vi "Read Record.vi"(8 "error in (no error)":errorcluster, 11 "Configuration Database Actor in":refnum<class "Configuration Database Actor.lvclass">) -> (0 "error out":errorcluster, 3 "Configuration Database Actor out":refnum<class "Configuration Database Actor.lvclass">)   [LabVIEW 2022 SP3, in "Configuration Database Actor.lvlib" / "Configuration Database Actor.lvclass"]
uses:
  Configuration Database Actor.lvclass
  C:/Program Files/National Instruments/LabVIEW 2022/vi.lib/ActorFramework/Actor/Actor.lvclass
  <vilib>/ActorFramework/Actor/Actor.lvclass/Actor.ctl
  Configuration Database Actor.lvclass/Configuration Database Actor.ctl
  Interface Elevator/Interface Elevator Messages/Read record from DB Msg/Read record from DB Msg.lvclass/Read record from DB Msg.ctl
  <vilib>/ActorFramework/Message Enqueuer/Message Enqueuer.lvclass/Message Enqueuer.ctl
  <vilib>/ActorFramework/Message Enqueuer/Enqueue.vi
  Interface Elevator/Interface Elevator Messages/Read record from DB Msg/Read record from DB Msg.lvclass
  C:/Program Files/National Instruments/LabVIEW 2022/vi.lib/ActorFramework/Message/Message.lvclass
  <vilib>/ActorFramework/Message Priority Queue/Priority Enqueue.vi
  <vilib>/ActorFramework/Actor/Actor.lvclass
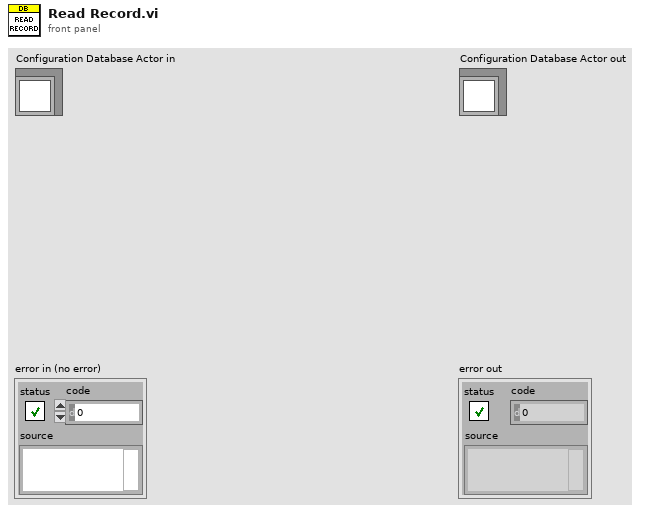
[diagram p1: front panel]
types:
  T1 = typedef "Configuration Database Actor.lvlib/Configuration Database Actor.lvclass/Record -Cluster.ctl" = cluster{"Door Open":dbl, "Door Close":dbl, "Travel Time":dbl, "Inactivity Time":dbl}
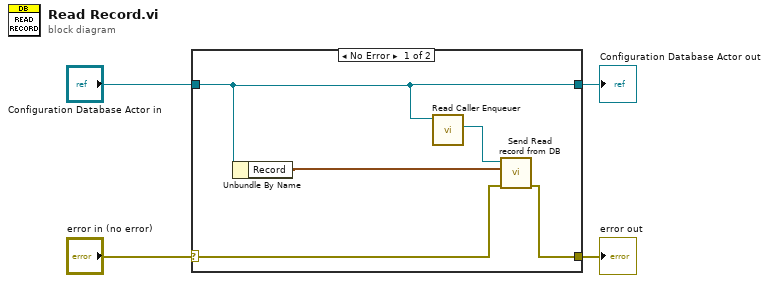
[diagram p0: block diagram]
diagram:
  n1 = case shown="No Error" "error in (no error)" {
    selector: "error in (no error)" -> [w7 w10]
    tunnel: [w6 w10] -> w3
    tunnel: [w9 w11] -> w1
    tunnel: "Configuration Database Actor in" -> [w9 w11]
    frame No Error {
      n2 = Unbundle By Name(w9) -> ("Record"=w5:T1)
      n3 = call <vilib>:"Read Caller Enqueuer.vi"("Actor"=w9) -> ("Caller Enqueuer"=w8:refnum<class "Message Enqueuer.lvclass">)  [unwired: 10 in]
      n4 = call "Send Read record from DB.vi"("error in (no error)"=w7, "Record"=w5, "Message Enqueuer"=w8) -> ("error out"=w6:errorcluster)  [unwired: 7 in, 1 out]
    }
    frame Error {
    }
  }
  "error out" <- w3
  "Configuration Database Actor out" <- w1
